vi "Shoulder Degree to Shoulder Angle.vi"(5 "Level Shoulder Enc Pos":dbl, 7 "Min Shoulder Enc Pos":dbl, 8 "Wanted Shoulder Angle (Degrees)":dbl) -> (2 "Target Shoulder Enc Pos":dbl)   [LabVIEW 2023]
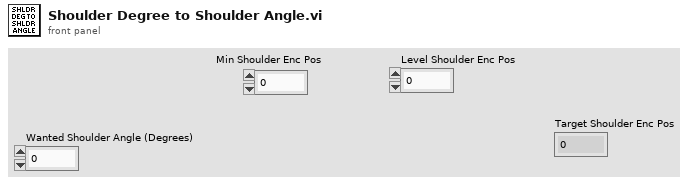
[diagram p1: front panel]
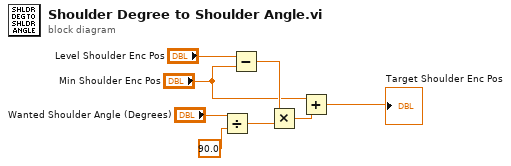
[diagram p0: block diagram]
diagram:
  n1 = Divide(x="Wanted Shoulder Angle (Degrees)", y=90.0) -> (x/y=w5:dbl)
  n2 = Subtract(x="Level Shoulder Enc Pos", y="Min Shoulder Enc Pos") -> (x-y=w4:dbl)
  n3 = Multiply(x=w4, y=w5) -> (x*y=w3:dbl)
  n4 = Add(x="Min Shoulder Enc Pos", y=w3) -> (x+y=→"Target Shoulder Enc Pos":dbl)
